vi "emi_Init GUI.vi"(9 "Change GUI background(T)":bool=TRUE, 11 "error in":errorcluster, 12 "Change graph backgrounds(T)":bool=TRUE, 13 "System background":T1={"Main Top Panels"={"Type"=enum."GlasGradBord 2", "Dark/Primary Color"=0, "Light/Secondary Color"=11776947, "Extra Color"=0}, "Main Botom Panels"={"Type"=enum."FlatColor", "Dark/Primary Color"=11776947, "Light/Secondary Color"=11776947, "Extra Color"=0}, "Graphs"={"Type"=enum."FlatColor", "Dark/Primary Color"=0, "Light/Secondary Color"=0, "Extra Color"=11776947}, "Dialogs"={"Type"=enum."FlatColor", "Dark/Primary Color"=16448250, "Light/Secondary Color"=16448250, "Extra Color"=0}}, 14 "Use Version info in Header(T)":bool=TRUE) -> (15 "error out":errorcluster)   [LabVIEW 2011]
doc: "Initialises a Sys01 GUI\n\nNotethat after this splash screen must be hidden, main window shown, settings collected and loops started.\n\nGets the size and position of main window(Where this VI is located) from default ini file.\nShows splash screen, \nmakes sure main window is hidden\nReinitialises all controls onmain window, \nSets Main windows background colors."
uses:
  Background/emi_System Colors.ctl
  Background/Private/_emi_ Color defenition.ctl
  Basic/0 - General/Graphix/Private/emi_List Of Graphix.ctl
  Profiling Mar-In/Splash & About/Private/emi_Splash&About Screen.vi
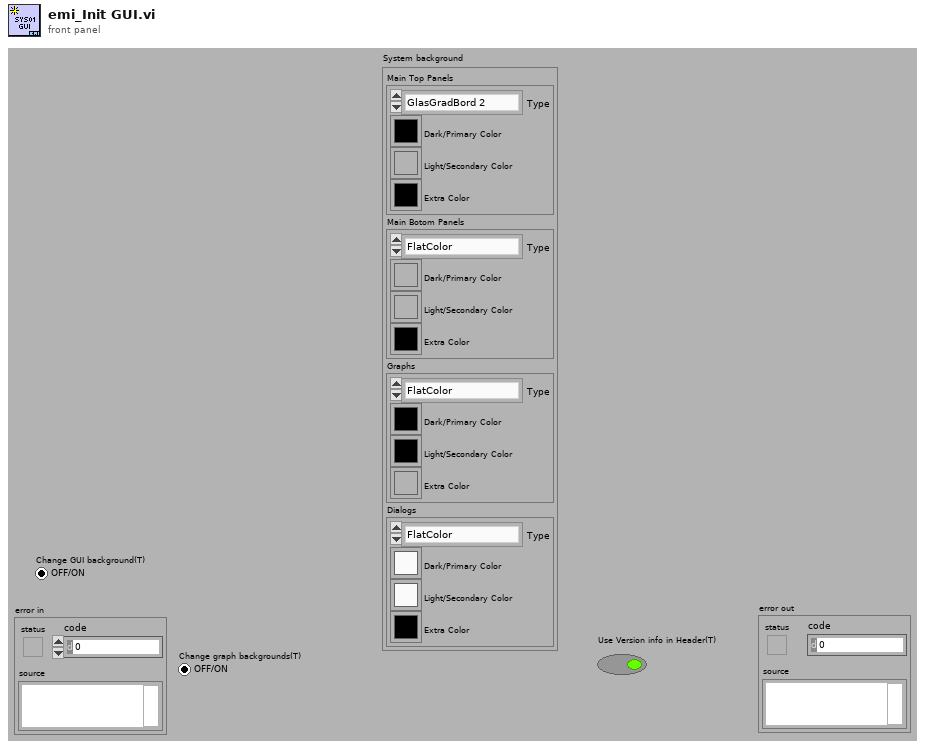
[diagram p1: front panel]
types:
  T1 = typedef "emi_System Colors.ctl" = cluster{"Main Top Panels":T2, "Main Botom Panels":T2, "Graphs":T2, "Dialogs":T2}
  T2 = typedef "_emi_ Color defenition.ctl" = cluster{"Type":T3, "Dark/Primary Color":u32, "Light/Secondary Color":u32, "Extra Color":u32}
  T3 = typedef "emi_List Of Graphix.ctl" = enum16{"FlatColor", "SharpGrad", "ShallowGrad", "GlasGradBord", "GlasGrad", "GlasGradBord 2"}
  T4 = enum32{"Invalid", "Standard", "Closed", "Hidden", "Minimized", "Maximized"}
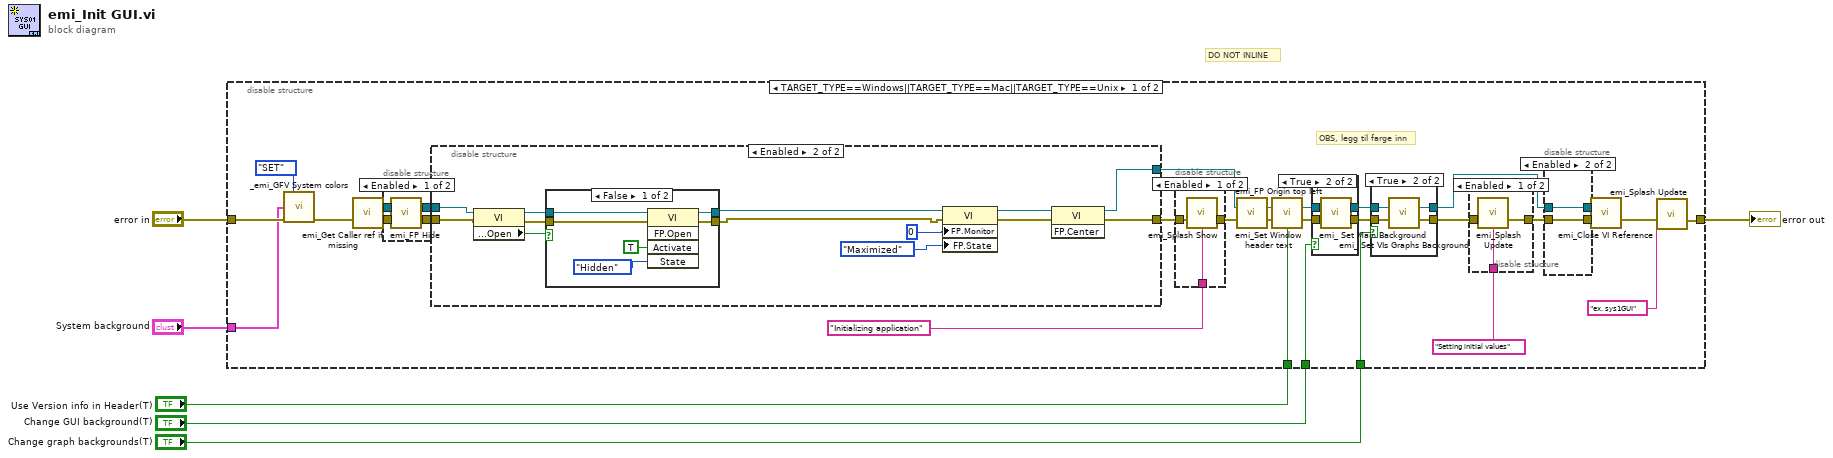
[diagram p0: block diagram]
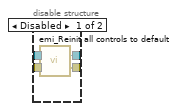
[diagram p6: hidden frame]
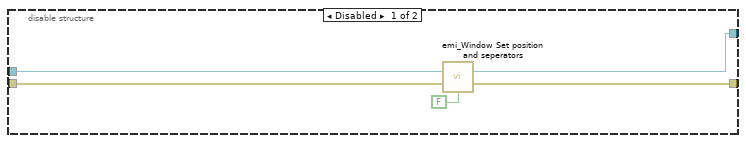
[diagram p7: hidden frame]
diagram:
  # "DO NOT INLINE"
  n1 = disable-structure shown="TARGET_TYPE==Windows||TARGET_TYPE==Mac||TARGET_TYPE==Unix" {
    disable-tunnel: "error in" -> [w26 w95]
    disable-tunnel: [w9 w95] -> w6
    disable-tunnel: "System background" -> [w24 _]
    disable-tunnel: "Change graph backgrounds(T)" -> [w14 _]
    disable-tunnel: "Use Version info in Header(T)" -> [w13 _]
    disable-tunnel: "Change GUI background(T)" -> [w7 _]
    frame condition #0 (active) {
      # "OBS, legg til farge inn"
      n2 = call "_emi_GFV System colors.vi"("Action(GET)"=enum16{"GET", "SET"}."SET", "System background in"=w24, "error in (no error)"=w26) -> ("error out"=w21:errorcluster)  [unwired: 11 in, 1 out]
      n3 = call "emi_Get Caller ref if missing.vi"("error in (no error)"=w21) -> ("VI Refnum Out"=w20:refnum<vi>, "error out"=w19:errorcluster)  [unwired: 12 in, 1 out]
      n4 = disable-structure shown="Enabled" {
        disable-tunnel: [w54 w56] -> w36
        disable-tunnel: w20 -> [w53 w55]
        disable-tunnel: w19 -> [w52 w56]
        disable-tunnel: [w51 w55] -> w12
        frame Enabled {
          n5 = call "emi_FP Hide.vi"("VI Refnum(This vi)"=w53, "error in (no error)"=w52) -> ("VI Refnum"=w51:refnum<vi>, "error out"=w54:errorcluster)  [unwired: 12 in]
        }
        frame Disabled {
        }
      }
      n6 = disable-structure shown="Enabled" {
        disable-tunnel: [w67 w76] -> w8
        disable-tunnel: w36 -> [w66 w71]
        disable-tunnel: w12 -> [w65 w70]
        disable-tunnel: [w64 w75] -> w34
        frame Disabled {
          n7 = call "emi_Window Set position and seperators.vi"("VI Refnum(This VI)"=w65, "error in (no error)"=w66, "Set Splitters(T)"=FALSE) -> ("VI Refnum"=w64:refnum<vi>, "error out"=w67:errorcluster)  [unwired: 11 in]
        }
        frame Enabled {
          n8 = property class="VI"(reference=w70, error in=w71) -> (reference out=w74:refnum<vi>, error out=w73:errorcluster, "Front Panel.Open"=w72:bool)
          n9 = case shown="False" w72 {
            tunnel: w73 -> [w85 w87]
            tunnel: w74 -> [w86 w88]
            tunnel: [w84 w87] -> w69
            tunnel: [w83 w88] -> w68
            frame False {
              n10 = invoke class="VI" method="FP.Open"(reference=w86, error in=w85, "Activate"=TRUE ("Activate?"), "State"=T4."Hidden") -> (reference out=w83:refnum<vi>, error out=w84:errorcluster)  [unwired: 1 in, 3 out]
            }
            frame True {
            }
          }
          n11 = property class="VI"(reference=w68, error in=w69, "FP.Monitor"=u16 0 ("Front Panel Window:Monitor"), "FP.State"=T4."Maximized" ("Front Panel Window:State")) -> (reference out=w77:refnum<vi>, error out=w78:errorcluster)
          n12 = invoke class="VI" method="FP.Center"(reference=w77, error in=w78) -> (reference out=w75:refnum<vi>, error out=w76:errorcluster)  [unwired: 1 in, 1 out]
        }
      }
      n13 = disable-structure shown="Enabled" {
        disable-tunnel: [w43 w44] -> w35
        disable-tunnel: "Initializing application" ("Status text") -> [w42 _]
        disable-tunnel: w8 -> [w41 w44]
        frame Enabled {
          n14 = call "emi_Splash Show.vi"("error In"=w41, "Status text"=w42) -> ("error out"=w43:errorcluster)  [unwired: 12 in, 1 out]
        }
        frame Disabled {
        }
      }
      n15 = call "emi_FP Origin top left.vi"("VI Refnum(This vi)"=w34, "error in (no error)"=w35) -> ("VI Refnum"=w31:refnum<vi>, "error out"=w32:errorcluster)  [unwired: 12 in]
      n16 = call "emi_Set Window header text.vi"("VI Refnum(This VI)"=w31, "error in (no error)"=w32, "Use Version info(F)"=w13) -> ("VI Refnum"=w22:refnum<vi>, "error out"=w23:errorcluster)  [unwired: 11 in]
      n17 = case shown="True" w7 {
        tunnel: w23 -> [w45 w50]
        tunnel: w22 -> [w46 w49]
        tunnel: [w45 w48] -> w18
        tunnel: [w46 w47] -> w16
        frame False {
        }
        frame True {
          n18 = call "emi_ Set Main Background.vi"("VI Refnum(This vi)"=w49, "error in (no error)"=w50) -> ("VI Refnum"=w47:refnum<vi>, "error out"=w48:errorcluster)  [unwired: 12 in]
        }
      }
      n19 = case shown="True" w14 {
        tunnel: w18 -> [w89 w94]
        tunnel: [w89 w93] -> w17
        tunnel: w16 -> [w90 w92]
        tunnel: [w90 w91] -> w15
        frame False {
        }
        frame True {
          n20 = call "emi_ Set VIs Graphs Background .vi"("VI Refnum(This vi)"=w92, "error in (no error)"=w94) -> ("VI Refnum"=w91:refnum<vi>, "error out"=w93:errorcluster)  [unwired: 12 in]
        }
      }
      n21 = disable-structure shown="Enabled" {
        disable-tunnel: "Setting initial values" ("Task Text") -> [w39 _]
        disable-tunnel: [w38 w40] -> w29
        disable-tunnel: w17 -> [w37 w40]
        frame Enabled {
          n22 = call "emi_Splash Update.vi"("error In"=w37, "Task Text"=w39) -> ("error out"=w38:errorcluster)  [unwired: 13 in]
        }
        frame Disabled {
        }
      }
      n23 = disable-structure shown="Enabled" {
        disable-tunnel: w29 -> [w60 w62]
        disable-tunnel: [w59 w62] -> w28
        disable-tunnel: [w58 w61] -> w27
        disable-tunnel: w15 -> [w57 w61]
        frame Disabled {
          n24 = call "emi_Reinit all controls to default.vi"("VI Refnum(This vi)"=w57, "error in (no error)"=w60) -> ("VI Refnum"=w58:refnum<vi>, "error out"=w59:errorcluster)  [unwired: 12 in]
        }
        frame Enabled {
        }
      }
      n25 = call "emi_Close VI Reference.vi"("VI Refnum"=w27, "error in (no error)"=w28) -> ("error out"=w10:errorcluster)  [unwired: 12 in, 1 out]
      n26 = call "emi_Splash Update.vi"("error In"=w10, "Task Text"="ex. sys1GUI") -> ("error out"=w9:errorcluster)  [unwired: 13 in]
    }
    frame condition #1 {
    }
  }
  "error out" <- w6
